vi "Calculate Check Sum.vi"(1 "String":string) -> (0 "String 2":string)   [LabVIEW 2009]
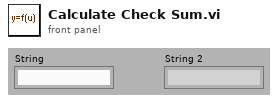
[diagram p1: front panel]
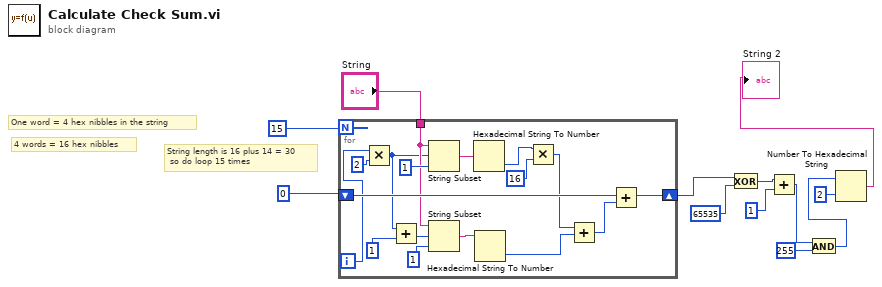
[diagram p0: block diagram]
diagram:
  # "One word = 4 hex nibbles in the string"
  # "4 words = 16 hex nibbles"
  # "String length is 16 plus 14 = 30\n so do loop 15 times"
  n1 = for {
    N: 15 -> [_]
    shift-right: [w13] -> w8
    shift-left: u8 0 -> [w27]
    tunnel: "String" -> [w26]
    i -> [w17]
    n2 = Multiply(x=w17, y=2) -> (x*y=w16:i32)
    n3 = Add(x=w16, y=i8 1) -> (x+y=w22:i32)
    n4 = String Subset(string=w26, offset (0)=w16, length (rest)=1) -> (substring=w28:string)
    n5 = String Subset(string=w26, offset (0)=w22, length (rest)=1 ("length (rest)")) -> (substring=w24:string)
    n6 = Hexadecimal String To Number(string=w28) -> (number=w20:u32)  [unwired: 2 in, 1 out]
    n7 = Hexadecimal String To Number(string=w24) -> (number=w15:u32)  [unwired: 2 in, 1 out]
    n8 = Multiply(x=w20, y=u32 16) -> (x*y=w14:u32)
    n9 = Add(x=w14, y=w15) -> (x+y=w21:u32)
    n10 = Add(x=w21, y=w27) -> (x+y=w13:u32)
  }
  n11 = Exclusive Or(1:u32 65535 ("y"), 2:w8) -> (0:w6:u32)
  n12 = Add(x=w6, y=u32 1) -> (x+y=w9:u32)
  n13 = And(x=w9, y=u32 255) -> (x .and. y?=w11:u32)
  n14 = Number To Hexadecimal String(1:i16 2 ("width (-)"), 2:w11) -> (0:→"String 2":string)
